vi "Get All Project Class Paths.vi"(8 "error in":errorcluster, 10 "Project File":path) -> (0 "error out":errorcluster, 2 "Project Classes":path[](array[path]))   [LabVIEW 2011, in "VITesterUtilities.lvlib"]
uses:
  Libraries/VITesterUtilities.lvlib
  C/Program Files (x86)/National Instruments/LabVIEW 2015/user.lib/_OpenG.lib/array/array.llb/Conditional Auto-Indexing Tunnel (String)__ogtk.vi
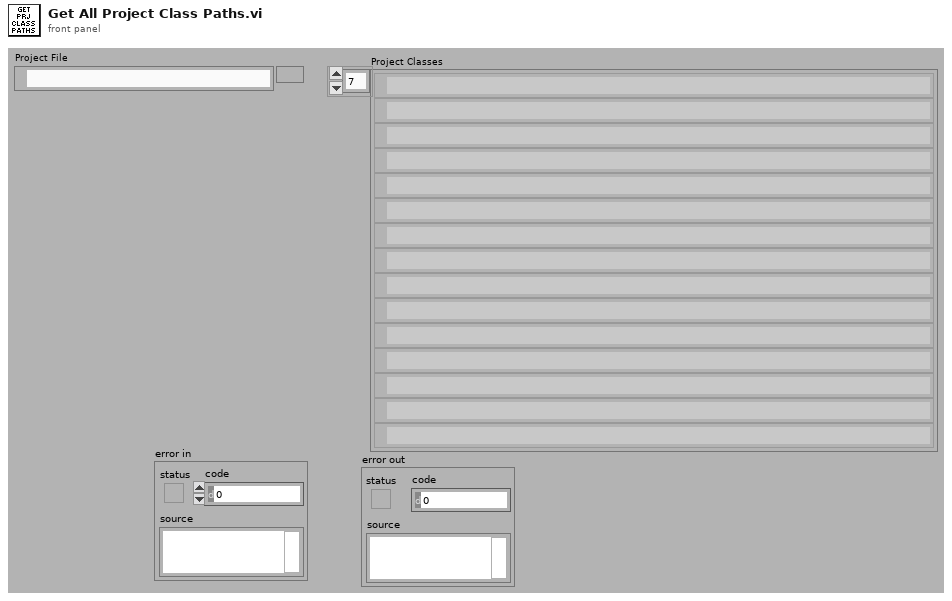
[diagram p1: front panel]
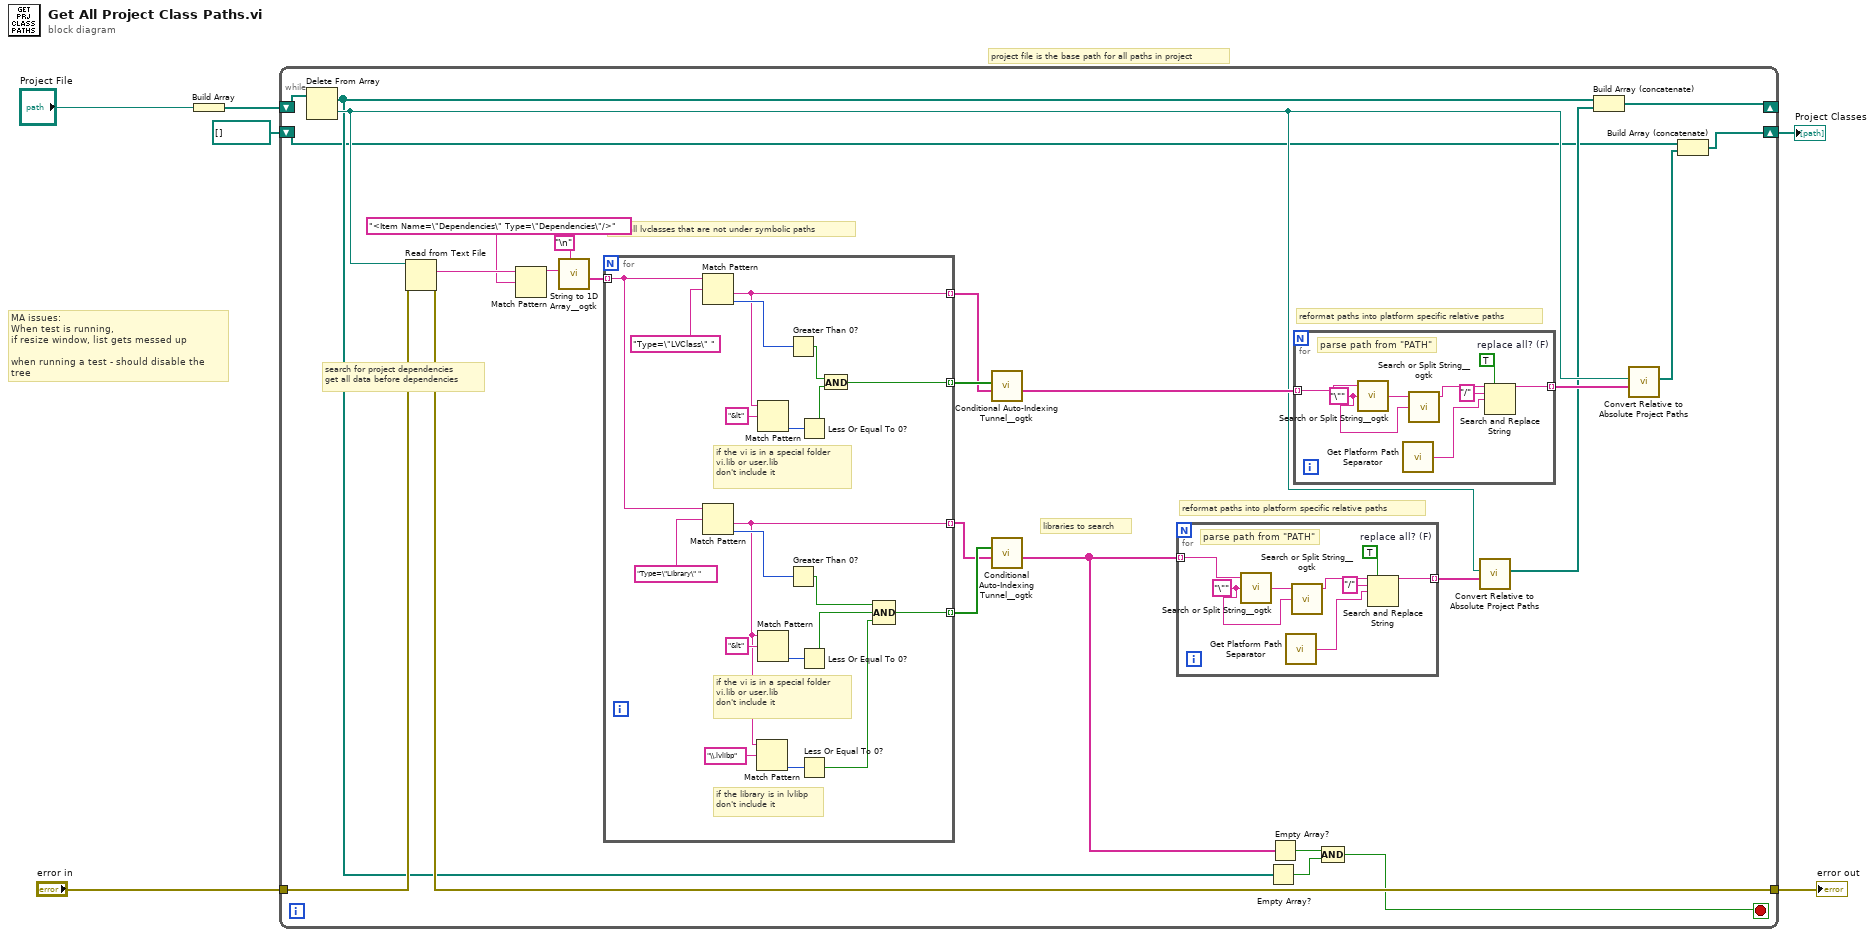
[diagram p0: block diagram]
diagram:
  # "MA issues:\nWhen test is running,\nif resize window, list gets messed up\n\nwhen running a test - should disable the tree"
  # "project file is the base path for all paths in project"
  n1 = Build Array("Project File") -> (w2:path[])
  n2 = while {
    tunnel: "error in" -> [w24]
    tunnel: [w23] -> w5
    shift-right: [w10] -> _
    shift-left: w2 -> [w16]
    shift-right: [w7] -> w4
    shift-left: path[] [] ("VI Absolute Paths") -> [w9]
    stop <- w13 stop-if-true
    # "reformat paths into platform specific relative paths"
    # "libraries to search"
    # "reformat paths into platform specific relative paths"
    # "find all lvclasses that are not under symbolic paths"
    # "search for project dependencies\nget all data before dependencies"
    n3 = Delete From Array(array=w16) -> (deleted portion=w15:path, array with subset deleted=w14:path[])  [unwired: 2 in]
    n4 = Read from Text File(file (use dialog)=w15, error in=w24) -> (text=w32:string, error out=w23:errorcluster)  [unwired: 2 in, 2 out]
    n5 = Match Pattern(string=w32, regular expression="<Item Name=\"Dependencies\" Type=\"Dependencies\"/>") -> (before substring=w30:string)  [unwired: 1 in, 3 out]
    n6 = call "String to 1D Array__ogtk.vi"("delimiter (Tab)"="\n", "string"=w30) -> ("Array of Strings"=w28:string[])  [unwired: 9 in]
    n7 = for {
      tunnel: w28 -> [w54] mode=indexing
      tunnel: [w61] -> w27 mode=indexing
      tunnel: [w66] -> w26 mode=indexing
      tunnel: [w52] -> w20 mode=indexing
      tunnel: [w53] -> w21 mode=indexing
      # "if the library is in lvlibp\ndon't include it"
      # "if the vi is in a special folder\nvi.lib or user.lib\ndon't include it"
      # "if the vi is in a special folder\nvi.lib or user.lib\ndon't include it"
      n8 = Match Pattern(string=w54, regular expression="Type=\"LVClass\" ") -> (after substring=w66:string, offset past match=w67:i32)  [unwired: 1 in, 2 out]
      n9 = Match Pattern(string=w54, regular expression="Type=\"Library\" ") -> (after substring=w52:string, offset past match=w56:i32)  [unwired: 1 in, 2 out]
      n10 = Match Pattern(string=w52, regular expression="\\.lvlibp") -> (offset past match=w50:i32)  [unwired: 1 in, 3 out]
      n11 = Match Pattern(string=w66, regular expression="&lt") -> (offset past match=w64:i32)  [unwired: 1 in, 3 out]
      n12 = Match Pattern(string=w52, regular expression="&lt") -> (offset past match=w58:i32)  [unwired: 1 in, 3 out]
      n13 = Greater Than 0?(x=w67) -> (x > 0?=w62:bool)
      n14 = Greater Than 0?(x=w56) -> (x > 0?=w60:bool)
      n15 = Less Or Equal To 0?(x=w64) -> (x <= 0?=w63:bool)
      n16 = Less Or Equal To 0?(x=w58) -> (x <= 0?=w59:bool)
      n17 = Less Or Equal To 0?(x=w50) -> (x <= 0?=w49:bool)
      n18 = And(x=w62, y=w63) -> (x .and. y?=w61:bool)
      n19 = Compound Arithmetic op=AND(w60, w59, w49) -> (w53:bool)
    }
    n20 = call-poly "Conditional Auto-Indexing Tunnel__ogtk.vi"("Array in"=w26, "Elements to keep"=w27) -> ("Filtered Array out"=w25:string[])  [unwired: 5 in]
    n21 = call-poly "Conditional Auto-Indexing Tunnel__ogtk.vi"("Array in"=w20, "Elements to keep"=w21) -> ("Filtered Array out"=w18:string[])  [unwired: 5 in]
    n22 = for {
      tunnel: w18 -> [w40] mode=indexing
      tunnel: [w34] -> w19 mode=indexing
      w33 = TRUE  # replace all? (F)
      w38 = "\"" ("search string/char (-)")
      # "parse path from \"PATH\""
      n23 = call "Search or Split String__ogtk.vi"("search string/char (-)"=w38, "string"=w40) -> ("substring after match"=w39:string)  [unwired: 1 in, 2 out]
      n24 = call "Get Platform Path Separator.vi"() -> ("platform path separator"=w36:string)
      n25 = call "Search or Split String__ogtk.vi"("search string/char (-)"=w38, "string"=w39) -> ("substring before match"=w35:string)  [unwired: 1 in, 2 out]
      n26 = Search and Replace String(replace all?=w33, input string=w35, search string="/", replace string=w36) -> (result string=w34:string)  [unwired: 4 in, 3 out]
    }
    n27 = Empty Array?(array=w14) -> (empty?=w12:bool)
    n28 = Empty Array?(array=w18) -> (empty?=w17:bool)
    n29 = for {
      tunnel: w25 -> [w48] mode=indexing
      tunnel: [w42] -> w22 mode=indexing
      w41 = TRUE  # replace all? (F)
      w46 = "\"" ("search string/char (-)")
      # "parse path from \"PATH\""
      n30 = call "Search or Split String__ogtk.vi"("search string/char (-)"=w46, "string"=w48) -> ("substring after match"=w47:string)  [unwired: 1 in, 2 out]
      n31 = call "Get Platform Path Separator.vi"() -> ("platform path separator"=w44:string)
      n32 = call "Search or Split String__ogtk.vi"("search string/char (-)"=w46, "string"=w47) -> ("substring before match"=w43:string)  [unwired: 1 in, 2 out]
      n33 = Search and Replace String(replace all?=w41, input string=w43, search string="/", replace string=w44) -> (result string=w42:string)  [unwired: 4 in, 3 out]
    }
    n34 = Compound Arithmetic op=AND(w17, w12) -> (w13:bool)
    n35 = call "Convert Relative to Absolute Project Paths.vi"("VI Relative Paths"=w19, "Project File"=w15) -> ("VI Absolute Paths"=w11:path[])  [unwired: 9 in]
    n36 = Build Array (concatenate)(w14, w11) -> (w10:path[])
    n37 = call "Convert Relative to Absolute Project Paths.vi"("VI Relative Paths"=w22, "Project File"=w15) -> ("VI Absolute Paths"=w8:path[])  [unwired: 9 in]
    n38 = Build Array (concatenate)(w9, w8) -> (w7:path[])
  }
  "Project Classes" <- w4
  "error out" <- w5
